vi "Lezeti_Power_Monitor_07.vi"() -> ()   [LabVIEW 2012]
uses:
  <vilib>/Utility/file.llb/Write To Spreadsheet File (DBL).vi
  <instrlib>/RIGOL DS1000 Series/Public/Data/Read (Multiple Waveforms).vi
  <instrlib>/RIGOL DS1000 Series/RIGOL DS1000 Series.lvlib
panel:
  in  "Channel 2":dbl
  out "Waveform Graph":waveform(dbl)[](graph)
  in  "Iteration Time":dbl
  in  "Timeout":dbl
  in  "Channel":dbl
  in  "stop":bool
  in  "VISA resource name":refnum<visa-resource-name>
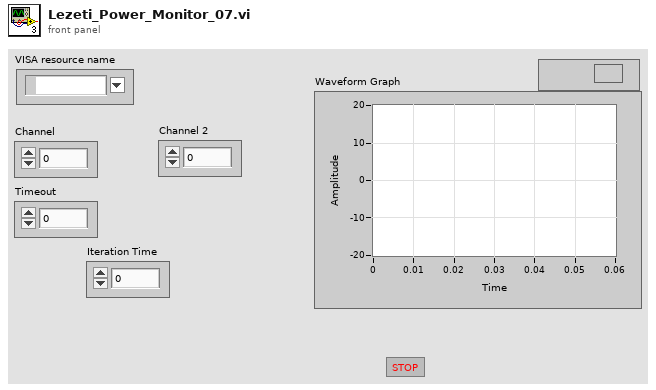
[diagram p1: front panel]
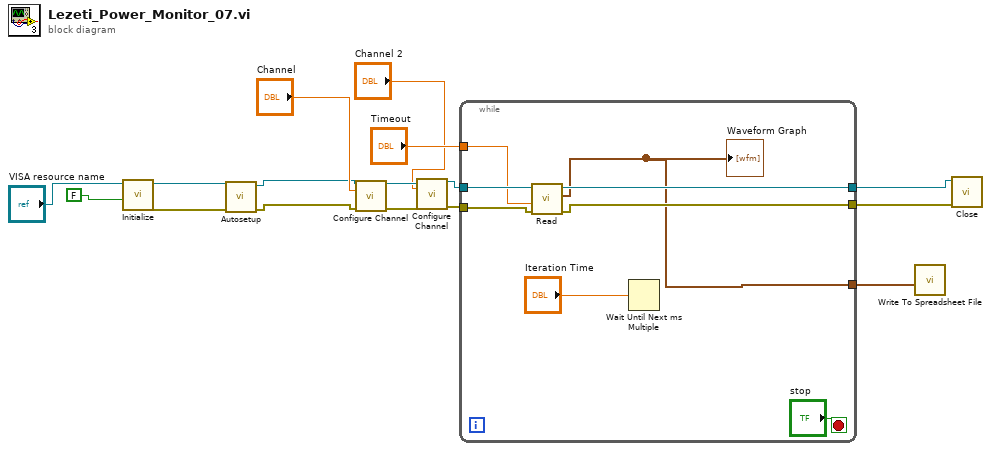
[diagram p0: block diagram]
diagram:
  n1 = call <instrlib>:"Initialize.vi"("Reset (True)"=FALSE, "VISA resource name"="VISA resource name") -> ("error out"=w3:errorcluster, "VISA resource name out"=w4:refnum<visa-resource-name>)  [unwired: 8 in]
  n2 = call <instrlib>:"Autosetup.vi"("error in (no error)"=w3, "VISA resource name"=w4) -> ("error out"=w1:errorcluster, "VISA resource name out"=w2:refnum<visa-resource-name>)  [unwired: 8 in]
  n3 = call <instrlib>:"Configure Channel.vi"("VISA resource name"=w2, "Channel (1: Channel 1)"="Channel", "error in (no error)"=w1) -> ("VISA resource name out"=w11:refnum<visa-resource-name>, "error out"=w10:errorcluster)  [unwired: 11 in]
  n4 = call <instrlib>:"Configure Channel.vi"("VISA resource name"=w11, "Channel (1: Channel 1)"="Channel 2", "error in (no error)"=w10) -> ("VISA resource name out"=w9:refnum<visa-resource-name>, "error out"=w8:errorcluster)  [unwired: 11 in]
  n5 = while {
    tunnel: w8 -> [w23]
    tunnel: w9 -> [w22]
    tunnel: [w21] -> w14
    tunnel: [w20] -> w13
    tunnel: "Timeout" -> [w19]
    tunnel: [w17] -> w5
    stop <- "stop" stop-if-true
    n6 = call-poly <instrlib>:"Read.vi"("error in (no error)"=w23, "Timeout (10000 ms)"=w19, "VISA resource name"=w22) -> ("error out"=w20:errorcluster, "Waveform Data"=w17:waveform(dbl)[], "VISA resource name out"=w21:refnum<visa-resource-name>)  [unwired: 6 in]
    "Waveform Graph" <- w17
    n7 = Wait Until Next ms Multiple(millisecond multiple="Iteration Time") -> ()  [unwired: 1 out]
  }
  n8 = call-poly <vilib>:"Write To Spreadsheet File.vi"("1D data"=w5) -> ()  [unwired: 7 in, 1 out]
  n9 = call <instrlib>:"Close.vi"("error in (no error)"=w13, "VISA resource name"=w14) -> ()  [unwired: 9 in, 1 out]
